vi "WritebyWeakRefI32Arr.vi"(8 "error in":errorcluster caption="entrée d'erreur", 10 "Valeur":i32[](array[numeric]), 11 "Control Ref":refnum<vi>) -> (0 "error out":errorcluster caption="sortie d'erreur")   [LabVIEW 2019]
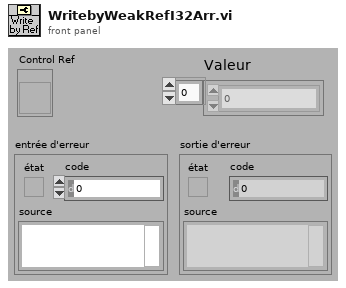
[diagram p1: front panel]
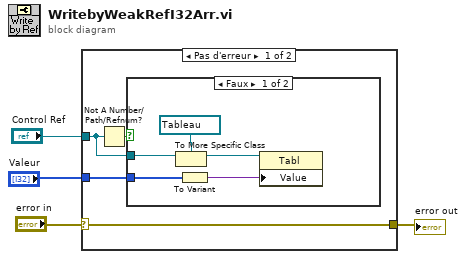
[diagram p0: block diagram]
diagram:
  n1 = case shown="Pas d'erreur" "error in" {
    selector: "error in" -> [w5 w14]
    tunnel: "Control Ref" -> [w7 _]
    tunnel: "Valeur" -> [w6 _]
    tunnel: [w5 w14] -> w2
    frame No Error {
      n2 = Not A Number/Path/Refnum?(number/path/refnum=w7) -> (NaN/Path/Refnum?=w8:bool)
      n3 = case shown="Faux" w8 {
        tunnel: w7 -> [w11 _]
        tunnel: w6 -> [w13 _]
        frame False {
          n4 = To More Specific Class(target class=refnum<vi> refnum ("référence"), reference=w11) -> (specific class reference=w10:refnum<vi>)  [unwired: 1 in, 1 out]
          n5 = To Variant(anything=w13) -> (Variant=w9:variant)
          n6 = property class="Tabl"(reference=w10, "Value"=w9) -> ()  [unwired: 1 in, 2 out]
        }
        frame True {
        }
      }
    }
    frame Error {
    }
  }
  "error out" <- w2
